vi "Plot Single Polar Point.vi"(6 "fill?(F)":bool, 7 "Size":i16, 8 "polar attributes":T2 {"minimum" format="%0.2f"; "maximum" format="%0.2f"}, 9 "grid measurements":T1 {"end angle" format="%0.2f"; "start angle" format="%0.2f"; "scale factors"."b" format="%0.2f"; "scale factors"."a" format="%0.2f"}, 10 "Polar Point":cluster{"magnitude":dbl, "phase":dbl} {"phase" format="%0.2f"; "magnitude" format="%0.2f"}, 11 "picture":picture) -> (3 "new picture":picture)   [LabVIEW 2012, in "Vector Function Generator.xctl"]
doc: "Original version modified by G. Burnell (g.burnell@leeds.ac.uk) for plotting on black background."
uses:
  Vector Function Generator.xctl
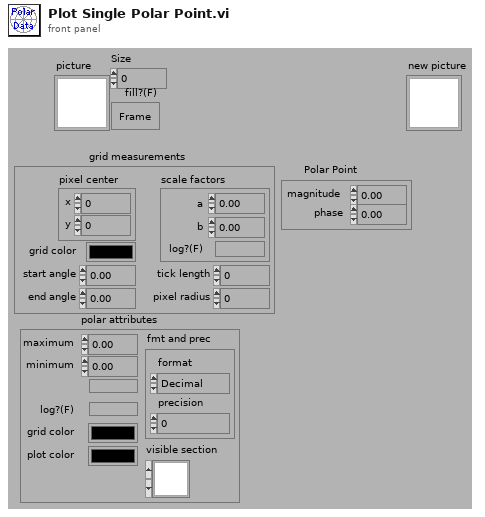
[diagram p1: front panel]
types:
  T1 = cluster{"pixel center":cluster{"x":i16, "y":i16}, "scale factors":cluster{"a":dbl, "b":dbl, "log?(F)":bool}, "grid color":u32, "start angle":dbl, "end angle":dbl, "tick length":i16, "pixel radius":i32}
  T2 = cluster{"maximum":dbl, "minimum":dbl, "clip to min":bool, "log?(F)":bool, "grid color":u32, "plot color":u32, "fmt and prec":cluster{"format":enum8{"Decimal", "Scientific", "Engineering", "Binary", "Octal", "Hex"}, "precision":u8}, "visible section":u16}
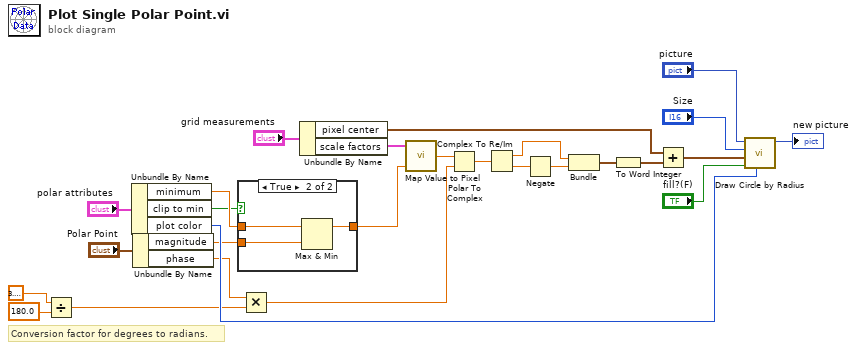
[diagram p0: block diagram]
diagram:
  # "Conversion factor for degrees to radians."
  n1 = Divide(x=3.141592653589793, y=180.0) -> (x/y=w15:dbl)
  n2 = Unbundle By Name("polar attributes") -> ("minimum"=w19:dbl, "clip to min"=w17:bool, "plot color"=w18:u32)
  n3 = Unbundle By Name("Polar Point") -> ("magnitude"=w5:dbl, "phase"=w3:dbl)
  n4 = case shown="True" w17 {
    tunnel: w5 -> [w28 w31]
    tunnel: [w28 w30] -> w6
    tunnel: w19 -> [_ w29]
    frame False {
    }
    frame True {
      n5 = Max & Min(x=w29, y=w31) -> (max(x,y)=w30:dbl)  [unwired: 1 out]
    }
  }
  n6 = Multiply(x=w3, y=w15) -> (x*y=w4:dbl)
  n7 = Unbundle By Name("grid measurements") -> ("pixel center"=w20:cluster{"x":i16, "y":i16}, "scale factors"=w21:cluster{"a":dbl, "b":dbl, "log?(F)":bool})
  n8 = call <vilib>:"Map Value to Pixel.vi"("x"=w6, "scale factors"=w21) -> ("pixel"=w7:dbl)  [unwired: 1 out]
  n9 = Polar To Complex(1:w4, 2:w7) -> (0:w13:cdb)
  n10 = Complex To Re/Im(x + iy=w13) -> (x=w11:dbl, y=w10:dbl)
  n11 = Negate(x=w10) -> (-x=w8:dbl)
  n12 = Bundle(w11, w8) -> (w12:cluster{dbl, dbl})  [unwired: 1 out]
  n13 = To Word Integer(number=w12) -> (16bit integer=w9:cluster{i16, i16})
  n14 = Add(x=w20, y=w9) -> (x+y=w24:cluster{i16, i16})
  n15 = call <vilib>:"Draw Circle by Radius.vi"("color(black)"=w18, "fill?(F)"="fill?(F)", "pixel center"=w24, "radius"="Size", "picture"="picture") -> ("new picture"=→"new picture":picture)  [unwired: 3 in, 3 out]
